vi "Single Tone Results to Cluster of Arrays.vi"(10 "results":T2[](array[typedef])) -> (2 "results (N chan)":T1)   [LabVIEW 2021]
uses:
  controls/single tone audio measurements.ctl
  controls/single tone audio measurements (N chan).ctl
  controls/audio controls.lvlib
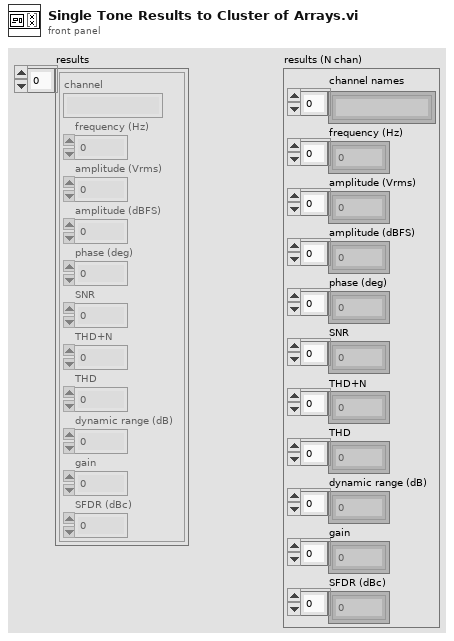
[diagram p1: front panel]
types:
  T1 = typedef "audio controls.lvlib/single tone audio measurements (N chan).ctl" = cluster{"channel names":string[], "frequency (Hz)":dbl[], "amplitude (Vrms)":dbl[], "amplitude (dBFS)":dbl[], "phase (deg)":dbl[], "SNR":dbl[], "THD+N":dbl[], "THD":dbl[], "dynamic range (dB)":dbl[], "gain":dbl[], "SFDR (dBc)":dbl[]}
  T2 = typedef "audio controls.lvlib/single tone audio measurements.ctl" = cluster{"channel":string, "frequency (Hz)":dbl, "amplitude (Vrms)":dbl, "amplitude (dBFS)":dbl, "phase (deg)":dbl, "SNR":dbl, "THD+N":dbl, "THD":dbl, "dynamic range (dB)":dbl, "gain":dbl, "SFDR (dBc)":dbl}
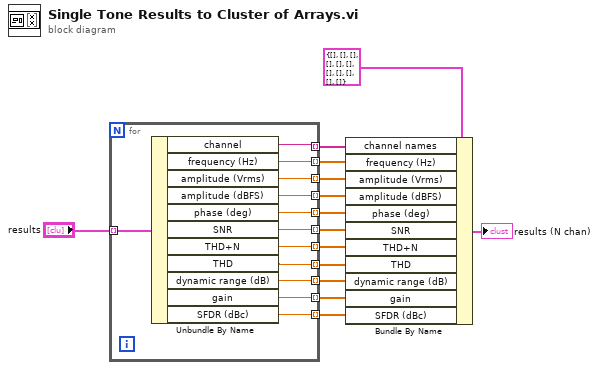
[diagram p0: block diagram]
diagram:
  n1 = for {
    tunnel: "results" -> [w26] mode=indexing
    tunnel: [w25] -> w12 mode=indexing
    tunnel: [w24] -> w11 mode=indexing
    tunnel: [w23] -> w10 mode=indexing
    tunnel: [w22] -> w9 mode=indexing
    tunnel: [w21] -> w8 mode=indexing
    tunnel: [w20] -> w7 mode=indexing
    tunnel: [w19] -> w6 mode=indexing
    tunnel: [w18] -> w5 mode=indexing
    tunnel: [w17] -> w4 mode=indexing
    tunnel: [w16] -> w3 mode=indexing
    tunnel: [w15] -> w2 mode=indexing
    n2 = Unbundle By Name(w26) -> ("channel"=w25:string, "frequency (Hz)"=w24:dbl, "amplitude (Vrms)"=w23:dbl, "amplitude (dBFS)"=w22:dbl, "phase (deg)"=w21:dbl, "SNR"=w20:dbl, "THD+N"=w19:dbl, "THD"=w18:dbl, "dynamic range (dB)"=w17:dbl, "gain"=w16:dbl, "SFDR (dBc)"=w15:dbl)
  }
  n3 = Bundle By Name(cluster=T1 {"channel names"=[], "frequency (Hz)"=[], "amplitude (Vrms)"=[], "amplitude (dBFS)"=[], "phase (deg)"=[], "SNR"=[], "THD+N"=[], "THD"=[], "dynamic range (dB)"=[], "gain"=[], "SFDR (dBc)"=[]} ("results"), "channel names"=w12, "frequency (Hz)"=w11, "amplitude (Vrms)"=w10, "amplitude (dBFS)"=w9, "phase (deg)"=w8, "SNR"=w7, "THD+N"=w6, "THD"=w5, "dynamic range (dB)"=w4, "gain"=w3, "SFDR (dBc)"=w2) -> (→"results (N chan)":T1)
